vi "Read Stop User Event.vi"(11 "Communication in":refnum<class "Communication.lvclass">) -> (2 "Stop User Event":refnum<user-event>)   [LabVIEW 2024, in "Communication.lvclass"]
uses:
  Communication.lvclass
  Communication.lvclass/Communication.ctl
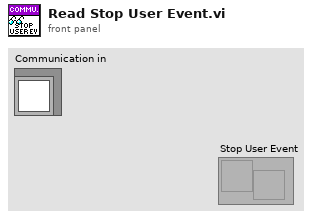
[diagram p1: front panel]
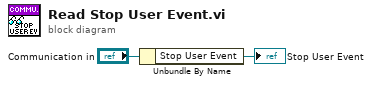
[diagram p0: block diagram]
diagram:
  n1 = Unbundle By Name("Communication in") -> ("Stop User Event"=→"Stop User Event":refnum<user-event>)
